vi "OFDM_BB.vi"() -> ()   [LabVIEW 2009]
uses:
  <vilib>/imath/engines/lvmath2/RunTimeEngine/ErrorHandling/NIMS_Finalize Error.vi
  <vilib>/imath/engines/lvmath2/RunTimeEngine/Parser/MC_Version.vi
  <vilib>/imath/engines/lvmath2/RunTimeEngine/NodeEndStatement/NIMS_NodeEndStatement_Output.vi
  <instcachedir>/0/NIMS_NodeEndStatement_Output_53EC0D466D134D7ABD903AC30B43404B.lvgen/NIMS_NodeEndStatement_Output_53EC0D466D134D7ABD903AC30B43404B_001.vi
  <instcachedir>/0/NIMS_NodeEndStatement_Output_53EC0D466D134D7ABD903AC30B43404B.lvgen/NIMS_NodeEndStatement_Output_53EC0D466D134D7ABD903AC30B43404B_002.vi
  <vilib>/imathl/engines/lvmath/Functions/Error Handling/Create Error.vi
  <vilib>/imath/engines/lvmath2/RunTimeEngine/ReplaceToken/NIMS_Replace - Assignment Check M(_,$)=VorM.vi
  <instcachedir>/0/NIMS_Replace - Assignment Check M(_,$)=VorM_3CB70357EF10473EBB509A04A4D02BC4.lvgen/NIMS_Replace - Assignment Check M(_,$)=VorM_3CB70357EF10473EBB509A04A4D02BC4_001.vi
  <vilib>/imath/engines/lvmath2/RunTimeEngine/ReplaceToken/NIMS_Replace - Size Check M(_,$)=VorM.vi
  <instcachedir>/0/NIMS_Replace - Size Check M(_,$)=VorM_EDDD90DB9294407A90551280BA264F99.lvgen/NIMS_Replace - Size Check M(_,$)=VorM_EDDD90DB9294407A90551280BA264F99_001.vi
  <vilib>/imath/engines/lvmath2/RunTimeEngine/ReplaceToken/NIMS_Replace - Check Row.vi
  <instcachedir>/0/NIMS_Replace - Check Row_C1FA588AB93341698A6951F0E3D02595.lvgen/NIMS_Replace - Check Row_C1FA588AB93341698A6951F0E3D02595_001.vi
  <vilib>/imath/engines/lvmath/Functions/Error Handling/MergeErrorsWrapper.vi
  <vilib>/imath/engines/lvmath/Functions/Error Handling/MC_Error Cluster From Error Code.vi
  <vilib>/imath/engines/lvmath2/RunTimeEngine/BuiltInFunctions/fft/NIMS_fft(GV).vi
  <instcachedir>/0/NIMS_fft(GV)_4C6467FC22F84E4BA42517A07EF978B0.lvgen/NIMS_fft(GV)_4C6467FC22F84E4BA42517A07EF978B0_000.vi
  <vilib>/imath/engines/lvmath2/RunTimeEngine/BuiltInFunctions/imag/NIMS_imag(Complex).vi
  <instcachedir>/0/NIMS_imag(Complex)_3180D40D00C843A49C2B33397F857BF3.lvgen/NIMS_imag(Complex)_3180D40D00C843A49C2B33397F857BF3_000.vi
panel:
  out "Sub carriers Imag":dbl[][](graph)
  out "Sub carriers Real":dbl[][](graph)
  out "Signal Time Domain":dbl[](graph)
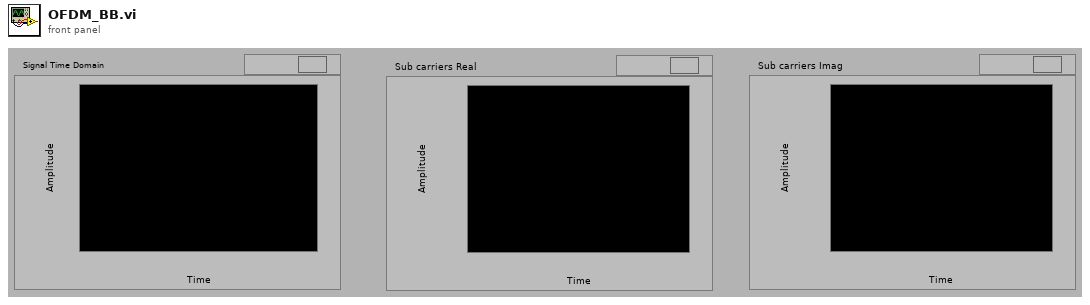
[diagram p1: front panel]
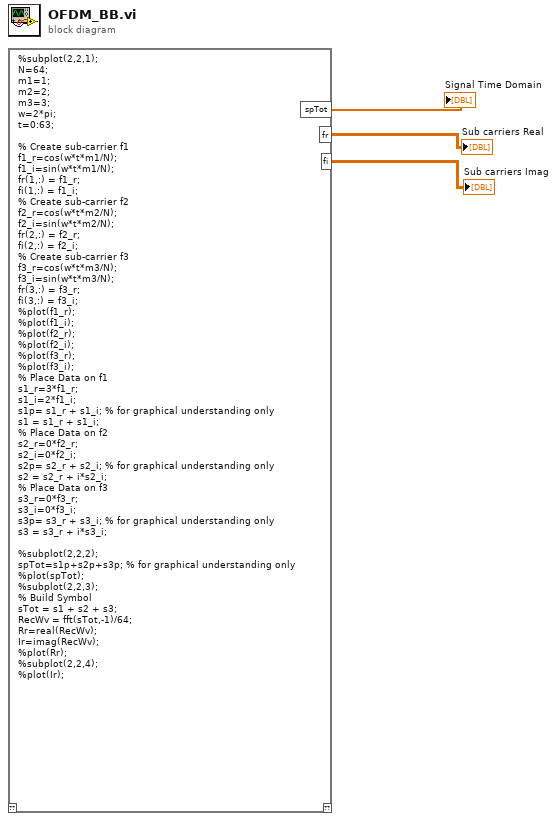
[diagram p0: block diagram]
diagram:
  n1 = mathscript code="%subplot(2,2,1);\nN=64;\nm1=1;\nm2=2;\nm3=3;\nw=2*pi;\nt=0:63;\n\n% Create sub-carrier f1\nf1_r=cos(w*t*m1/N);\nf1_i=sin(w*t*m1/N);\nfr(1,:) = f1_r;\nfi(1,:) = f1_i;\n% Create sub-carrier f2\nf2_r=cos(w*t*m2/N);\nf2_i=sin(w*t*m2/N);\nfr(2,:) = f2_r;\nfi(2,:) = f2_i;\n% Create sub-carrier f3\nf3_r=cos(w*t*m3/N);\nf3_i=sin(w*t*m3/N);\nfr(3,:) = f3_r;\nfi(3,:) = f3_i;\n%plot(f1_r);\n%plot(f1_i);\n%plot(f2_r);\n%plot(f2_i);\n%plot(f3_r);\n%plot(f3_i);\n% Place Data on f1\ns1_r=3*f1_r;\ns1_i=2*f1_i;\ns1p= s1_r + s1_i; % for graphical understanding only\ns1 = s1_r + s1_i;\n% Place Data on f2\ns2_r=0*f2_r;\ns2_i=0*f2_i;\ns2p= s2_r + s2_i; % for graphical understanding only\ns2 = s2_r + i*s2_i;\n% Place Data on f3\ns3_r=0*f3_r;\ns3_i=0*f3_i;\ns3p= s3_r + s3_i; % for graphical understanding only\ns3 = s3_r + i*s3_i;\n\n%subplot(2,2,2);\nspTot=s1p+s2p+s3p; % for graphical understanding only\n%plot(spTot);\n%subplot(2,2,3);\n% Build Symbol\nsTot = s1 + s2 + s3;\nRecWv = fft(sTot,-1)/64;\nRr=real(RecWv);\nIr=imag(RecWv);\n%plot(Rr);\n%subplot(2,2,4);\n%plot(Ir);"() -> ("spTot"=→"Signal Time Domain":dbl[], "fr"=→"Sub carriers Real":dbl[][], "fi"=→"Sub carriers Imag":dbl[][])  [unwired: 1 in, 1 out]
